vi "Close.vi"(8 "error in (no error)":errorcluster, 11 "reference":refnum<k24>) -> (0 "error out":errorcluster)   [LabVIEW 2017, in "piezojena NV40Single.lvlib"]
doc: "Close <b>reference</b> if it is a valid RefNum.\nEven if <b>error in</b> is an error, Dispose is called before closing the <b>reference</b>."
uses:
  piezojena NV40Single.lvlib
  C:/Users/Spenser Burrows/Desktop/Work/Labview software for spectrometer/PiezoStage_John/Piezojena.Protocols.Nv40Single.dll
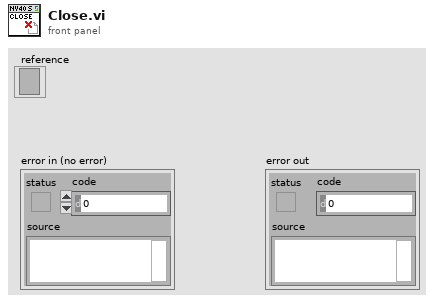
[diagram p1: front panel]
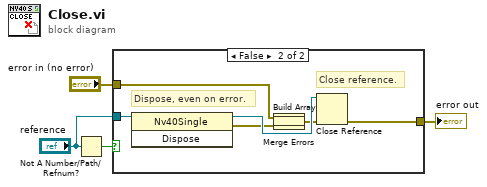
[diagram p0: block diagram]
diagram:
  n1 = Not A Number/Path/Refnum?(number/path/refnum="reference") -> (NaN/Path/Refnum?=w1:bool)
  n2 = case shown="False" w1 {
    tunnel: [w5 w11] -> w4
    tunnel: "reference" -> [_ w10]
    tunnel: "error in (no error)" -> [w5 w7]
    frame True {
      # "reference is not valid"
    }
    frame False {
      # "Close reference."
      # "Dispose, even on error."
      n3 = invoke class="Nv40Single" method="Dispose"(reference=w10) -> (reference out=w12:refnum<k24>, error out=w9:errorcluster)  [unwired: 2 in, 1 out]
      n4 = Build Array(w7, w9) -> (w6:errorcluster[])
      n5 = Merge Errors(w6) -> (w8:errorcluster)
      n6 = Close Reference(reference=w12, error in (no error)=w8) -> (error out=w11:errorcluster)
    }
  }
  "error out" <- w4
